vi "MillisecondsToWait.vi"(0 "milliseconds to wait":dbl format="%.3f") -> ()   [LabVIEW 2013]
uses:
  NI_Timer.dll
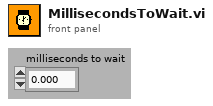
[diagram p1: front panel]
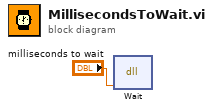
[diagram p0: block diagram]
diagram:
  n1 = dll-call lib="C:/Users/HamiltonDesignAir/Documents/~LabVIEW Archive/LabVIEW Programming Resource/High Resolution Timer/NI_Timer.dll" fn="Wait"("wait"="milliseconds to wait") -> ()  [unwired: 5 in, 2 out]
